vi "断电保存全局.vi"() -> ()   [LabVIEW 2016]
panel:
  out "线程":bool[](array[boolean])
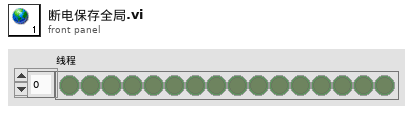
[diagram p1: front panel]
diagram:
